vi "separate_led_data.vi"(10 "Data from Stream":cluster{"LED1?":bool, "Data":dbl}[](array[cluster])) -> (1 "LED2":dbl[](array[numeric]), 2 "LED1":dbl[](array[numeric]))   [LabVIEW 2014]
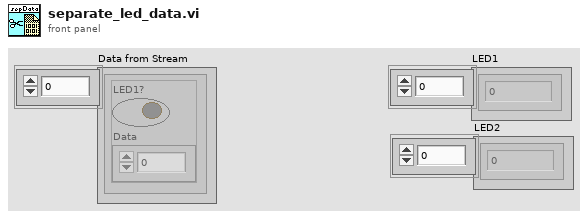
[diagram p1: front panel]
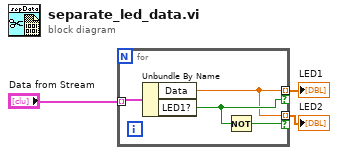
[diagram p0: block diagram]
diagram:
  n1 = for {
    tunnel: "Data from Stream" -> [w7] mode=indexing
    tunnel: [w5] -> w2 mode=indexing if=w6
    tunnel: [w5] -> w1 mode=indexing if=w4
    n2 = Unbundle By Name(w7) -> ("Data"=w5:dbl, "LED1?"=w6:bool)
    n3 = Not(x=w6) -> (.not. x?=w4:bool)
  }
  "LED1" <- w2
  "LED2" <- w1
